vi "get_spnial_column_MD5.vi"(11 "spinal_column":T1={"Experimental Variables"={"Pixel Size before binning (µm)"=0.0, "Imaging Wavelength (m)"=0.0, "Isotope"=0, "1P1 Linewidth (MHz)"=0.0, "Imaging Detuning (MHz)"=0.0, "Software Bin Size"=0, "Exp. Trigger ON time (ms)"=0.0, "Path to spinapi.dll"=path "C:/SpinCore/SpinAPI/lib32/spinapi.dll", "PB clock_freq (MHz)"=100.0}, "Red MOT 88 Inputs"={"Active Device"="", "Active Channels"=[], "Waveform Parameters"=[], "Active Phases"=[], "Phase Times"=[], "Trigger Channel"=""}, "6713 Blue MOT"={"Active Device"="", "Active Channels"=[], "Waveform Parameters"=[], "Active Phases"=[], "Phase Times"=[], "Trigger Channel"="", "FIFO Buffer Size"=0.0, "6713_ch_labels"={"Array"=["", "", "", "", "", "", "", "", "", "", "", "", "", "", "", "", "", "", "", "", " ", "", "", ""], "PB_0_Ch_Labels\n"=["0", "1", "2", "3", "4", "5", "6", "7", "8", "9", "10", "11", "12", "13", "14", "15", "16", "17", "18", "19", "20", "21", "22", "23"]}}, "48ch_pb_array"=[], "Red MOT 87 Inputs"={"Active Device"="", "Active Channels"=[], "Waveform Parameters"=[], "Active Phases"=[], "Phase Times"=[], "Trigger Channel"=""}, "ODT Params"={"Waveform Parameters"=[], "Active Phases"=[], "Active Channels"=[], "Phase Times (s)"=[], "Active Device"="", "Trigger Channel"="", "Evaporation Phase"=0.0, "Evaporation Channel"=0.0}, "Agilent E3631A Settings"={"VISA resource name"="", "Voltage Set (6V max)"=0.0, "Current Set (5A max)"=0.0, "Voltage Set (25V max)"=0.0, "Current Set (1A max)"=0.0, "Voltage Set (-25V max)"=25.0, "Current Set (1A max)"=0.225, "6V Switch"=FALSE, "+25V Switch"=FALSE, "-25V Switch"=FALSE, "Agilent E3631A Measurements"={"6V Actual Voltage Level (V)"=0.03231557, "6V Actual Current Level (A)"=0.01701259, "25V Actual Voltage Level (V)"=0.4256878, "25V Actual Current Level (A)"=0.2772881, "-25V Actual Current Level (A)"=0.0, "-25V Actual Voltage Level (V)"=0.0}, "Triggered Agilent Settings"={"Trigger \nDelay (s)"=3.0, "Enable +6V Channel"=TRUE, "+6V Current"=0.02, "Enable -25V Channel"=FALSE, "-25V Current"=0.0, "Enable +25V Channel"=TRUE, "+25V Current"=0.275}, "Auto Program Agilent"=FALSE, "Agilent Software Trigger"=FALSE}, "PixelFly Controls"={"Acquitsition Settings"={"Buffer number"=0, "Size (Bytes)"=0, "initialized array"=array2048x1280[2621440 elements], "X Bin"=0, "Y Bin"=0, "Board Handle"=0, "Picture parameters"={"ccdxsize"=0, "ccdy"=0, "pictx"=0, "picty"=0, "bitspixel"=12}, "Buffer Out"=[]}, "Initialization"={"Exposure mode"=1, "exp time"=150, "exp level"=1, "gain"=0, "boardid in"=0, "offset"=0, "V bin"=0, "H bin"=0, "trigger"=FALSE, "Bit depth"=0}}, "Scan Parameters"={"Initial Values"=[], "Final Values"=[], "Step Sizes"=[], "Parameters to Change"=[], "Channels to Change"=[], "Number of Parameters to Scan"=0, "Parameter Nickname (no spaces)"=[], "Scan Base Name"="", "Raw_Data Folder"=path "", "ROI Parameters"={"Background Radius"=0.0, "Atom Radius"=0.0, "X Center"=0.0, "Y Center"=0.0}, "Drop Time (ms)"=0.0, "Phases To Change"=[], "Scan Pulseblaster Channel With Parameter"={"Change PB Time Toggle"=FALSE, "PB Channel"=0.0, "Parameter Number"=0.0}, "Preserve Waveform\nContinuity"=FALSE, "Generated Array Type"=enum."Custom Array From File", "Master Batch Third Column"=0.0, "Master Batch Fourth Column"=0.0, "Master Batch Fifth Column"=0.0, "Current Param. Values"=[81.5, 1.0]}, "PicoScope"={"Channel A Settings"={"Enabled"=FALSE, "Coupling"=0, "Range"=0, "Analogue Offset"=0.0}, "Channel B Settings"={"Enabled"=FALSE, "Coupling"=0, "Range"=0, "Analogue Offset"=0.0}, "Trigger Options"={"Trigger Enabled"=FALSE, "Trigger Source"=enum."Channel A", "Trigger Threshold (-5 to 5 V)"=0.0, "Trigger Slope"=0, "Trigger Delay (s)"=0.0, "Auto Trigger Time (ms)"=0}, "Pico Scope Inititalization Settings"={"USB Power"=FALSE, "Use Serial Number"=FALSE, "Resolution"=0, "Serial Number"="", "Handle"=0}, "Use PicoScope?"=FALSE, "Acquisition Settings"={"Pre Trigger Time (s)"=0.0, "Post Trigger Time (s)"=0.0, "Resolution (s)"=0.0, "Four Channel Device"=FALSE, "Number of Captures"=0.0}}, "6229 Green Lattice Inputs"={"Active Device"="", "Active Channels"=[], "Active Phases"=[], "Phase Times"=[], "Trigger Channel"="", "FIFO Buffer Size"=0.0, "Sample Step Time (us)"=0.0, "Initialization Parameters"={"Enable Initialization"=FALSE, "Initial Values"=[]}, "Waveform Parameters"=[]}, "Novatech Synth Settings"=[], "Control Reference Cluster"={"Controls[]"=[], "Control Names"=[]}, "FPGA_cntrl"={"Channel 0"={"Operation"=0, "Input A"=0, "Output - LO"=0.0, "Output - HI"=0.0, "Inputs"=[0, 0, 0, 0], "Output Values"=[0.0, 0.0, 0.0, 0.0, 0.0], "Num. Inputs"=0, "Set Point"=0.0, "Inv."=[FALSE, FALSE, FALSE, FALSE], "Inv. A"=FALSE, "Inv. B"=FALSE, "Input B"=0}, "Channel 1"={"Operation"=0, "Input A"=0, "Output - LO"=0.0, "Output - HI"=0.0, "Inputs"=[0, 0, 0, 0], "Output Values"=[0.0, 0.0, 0.0, 0.0, 0.0], "Num. Inputs"=0, "Set Point"=0.0, "Inv."=[FALSE, FALSE, FALSE, FALSE], "Inv. A"=FALSE, "Inv. B"=FALSE, "Input B"=0}, "Channel 2"={"Operation"=0, "Input A"=0, "Output - LO"=0.0, "Output - HI"=0.0, "Inputs"=[0, 0, 0, 0], "Output Values"=[0.0, 0.0, 0.0, 0.0, 0.0], "Num. Inputs"=0, "Set Point"=0.0, "Inv."=[FALSE, FALSE, FALSE, FALSE], "Inv. A"=FALSE, "Inv. B"=FALSE, "Input B"=0}, "Channel 3"={"Operation"=0, "Input A"=0, "Output - LO"=0.0, "Output - HI"=0.0, "Inputs"=[0, 0, 0, 0], "Output Values"=[0.0, 0.0, 0.0, 0.0, 0.0], "Num. Inputs"=0, "Set Point"=0.0, "Inv."=[FALSE, FALSE, FALSE, FALSE], "Inv. A"=FALSE, "Inv. B"=FALSE, "Input B"=0}, "Channel 4"={"Operation"=0, "Input A"=0, "Output - LO"=0.0, "Output - HI"=0.0, "Inputs"=[0, 0, 0, 0], "Output Values"=[0.0, 0.0, 0.0, 0.0, 0.0], "Num. Inputs"=0, "Set Point"=0.0, "Inv."=[FALSE, FALSE, FALSE, FALSE], "Inv. A"=FALSE, "Inv. B"=FALSE, "Input B"=0}, "Channel 5"={"Operation"=0, "Input A"=0, "Output - LO"=0.0, "Output - HI"=0.0, "Inputs"=[0, 0, 0, 0], "Output Values"=[0.0, 0.0, 0.0, 0.0, 0.0], "Num. Inputs"=0, "Set Point"=0.0, "Inv."=[FALSE, FALSE, FALSE, FALSE], "Inv. A"=FALSE, "Inv. B"=FALSE, "Input B"=0}, "Channel 6"={"Operation"=0, "Input A"=0, "Output - LO"=0.0, "Output - HI"=0.0, "Inputs"=[0, 0, 0, 0], "Output Values"=[0.0, 0.0, 0.0, 0.0, 0.0], "Num. Inputs"=0, "Set Point"=0.0, "Inv."=[FALSE, FALSE, FALSE, FALSE], "Inv. A"=FALSE, "Inv. B"=FALSE, "Input B"=0}, "Channel 7"={"Operation"=0, "Input A"=0, "Output - LO"=0.0, "Output - HI"=0.0, "Inputs"=[0, 0, 0, 0], "Output Values"=[0.0, 0.0, 0.0, 0.0, 0.0], "Num. Inputs"=0, "Set Point"=0.0, "Inv."=[FALSE, FALSE, FALSE, FALSE], "Inv. A"=FALSE, "Inv. B"=FALSE, "Input B"=0}, "Channel 8"={"Operation"=0, "Input A"=0, "Output - LO"=0.0, "Output - HI"=0.0, "Inputs"=[0, 0, 0, 0], "Output Values"=[0.0, 0.0, 0.0, 0.0, 0.0], "Num. Inputs"=0, "Set Point"=0.0, "Inv."=[FALSE, FALSE, FALSE, FALSE], "Inv. A"=FALSE, "Inv. B"=FALSE, "Input B"=0}, "Channel 9"={"Operation"=0, "Input A"=0, "Output - LO"=0.0, "Output - HI"=0.0, "Inputs"=[0, 0, 0, 0], "Output Values"=[0.0, 0.0, 0.0, 0.0, 0.0], "Num. Inputs"=0, "Set Point"=0.0, "Inv."=[FALSE, FALSE, FALSE, FALSE], "Inv. A"=FALSE, "Inv. B"=FALSE, "Input B"=0}, "Channel 10"={"Operation"=0, "Input A"=0, "Output - LO"=0.0, "Output - HI"=0.0, "Inputs"=[0, 0, 0, 0], "Output Values"=[0.0, 0.0, 0.0, 0.0, 0.0], "Num. Inputs"=0, "Set Point"=0.0, "Inv."=[FALSE, FALSE, FALSE, FALSE], "Inv. A"=FALSE, "Inv. B"=FALSE, "Input B"=0}, "Channel 11"={"Operation"=0, "Input A"=0, "Output - LO"=0.0, "Output - HI"=0.0, "Inputs"=[0, 0, 0, 0], "Output Values"=[0.0, 0.0, 0.0, 0.0, 0.0], "Num. Inputs"=0, "Set Point"=0.0, "Inv."=[FALSE, FALSE, FALSE, FALSE], "Inv. A"=FALSE, "Inv. B"=FALSE, "Input B"=0}, "Channel 12"={"Operation"=0, "Input A"=0, "Output - LO"=0.0, "Output - HI"=0.0, "Inputs"=[0, 0, 0, 0], "Output Values"=[0.0, 0.0, 0.0, 0.0, 0.0], "Num. Inputs"=0, "Set Point"=0.0, "Inv."=[FALSE, FALSE, FALSE, FALSE], "Inv. A"=FALSE, "Inv. B"=FALSE, "Input B"=0}, "Channel 13"={"Operation"=0, "Input A"=0, "Output - LO"=0.0, "Output - HI"=0.0, "Inputs"=[0, 0, 0, 0], "Output Values"=[0.0, 0.0, 0.0, 0.0, 0.0], "Num. Inputs"=0, "Set Point"=0.0, "Inv."=[FALSE, FALSE, FALSE, FALSE], "Inv. A"=FALSE, "Inv. B"=FALSE, "Input B"=0}, "Channel 14"={"Operation"=0, "Input A"=0, "Output - LO"=0.0, "Output - HI"=0.0, "Inputs"=[0, 0, 0, 0], "Output Values"=[0.0, 0.0, 0.0, 0.0, 0.0], "Num. Inputs"=0, "Set Point"=0.0, "Inv."=[FALSE, FALSE, FALSE, FALSE], "Inv. A"=FALSE, "Inv. B"=FALSE, "Input B"=0}, "Channel 15"={"Operation"=0, "Input A"=0, "Output - LO"=0.0, "Output - HI"=0.0, "Inputs"=[0, 0, 0, 0], "Output Values"=[0.0, 0.0, 0.0, 0.0, 0.0], "Num. Inputs"=0, "Set Point"=0.0, "Inv."=[FALSE, FALSE, FALSE, FALSE], "Inv. A"=FALSE, "Inv. B"=FALSE, "Input B"=0}}} {"Experimental Variables"."Software Bin Size" items=["1"=1, "2"=2, "3"=3, "4"=4, "5"=5, "6"=6, "7"=7, "8"=8]; "Experimental Variables"."Isotope" min=84 max=88; "Experimental Variables"."Imaging Wavelength (m)" format="%#_6p"; "Red MOT 88 Inputs"."Phase Times" format="%.0p"; "Red MOT 88 Inputs"."Waveform Parameters"."Degree" min=1.0; "6713 Blue MOT"."Phase Times" format="%.3f"; "48ch_pb_array"."Label and Instructions"."Instruct Data" format="%#.2p"; "48ch_pb_array"."Label and Instructions"."Op Code" items=["Continue", "Stop", "Loop", "End Loop", "JSR", "RTS", "Go To", "Long Delay", "Wait"]; "48ch_pb_array"."Label and Instructions"."Time (s)" min=5e-08 format="%.2p"; "Red MOT 87 Inputs"."Phase Times" format="%.0p"; "Red MOT 87 Inputs"."Waveform Parameters"."Degree" min=1.0; "ODT Params"."Evaporation Channel" min=0.0 max=1.0 step=1.0; "ODT Params"."Evaporation Phase" min=0.0 max=4.0 step=1.0; "ODT Params"."Phase Times (s)" format="%#_6p"; "Agilent E3631A Settings"."Triggered Agilent Settings"."Trigger \nDelay (s)" min=0.0 max=3600.0 step=1.0 format="%.2f"; "Agilent E3631A Settings"."Agilent E3631A Measurements"."-25V Actual Current Level (A)" format="%.3g"; "Agilent E3631A Settings"."Agilent E3631A Measurements"."-25V Actual Voltage Level (V)" format="%.3g"; "Agilent E3631A Settings"."Agilent E3631A Measurements"."25V Actual Current Level (A)" format="%.3g"; "Agilent E3631A Settings"."Agilent E3631A Measurements"."25V Actual Voltage Level (V)" format="%.3g"; "Agilent E3631A Settings"."Agilent E3631A Measurements"."6V Actual Current Level (A)" format="%.3g"; "Agilent E3631A Settings"."Agilent E3631A Measurements"."6V Actual Voltage Level (V)" format="%.3g"; "Agilent E3631A Settings"."Current Set (1A max)" format="%.3g"; "Agilent E3631A Settings"."Voltage Set (-25V max)" format="%.3g"; "Agilent E3631A Settings"."Current Set (1A max)" format="%.3g"; "Agilent E3631A Settings"."Voltage Set (25V max)" format="%.3g"; "Agilent E3631A Settings"."Current Set (5A max)" format="%.3g"; "Agilent E3631A Settings"."Voltage Set (6V max)" format="%.3g"; "PixelFly Controls"."Initialization"."Bit depth" items=["8", "12"]; "PixelFly Controls"."Initialization"."H bin" items=["1", "2"]; "PixelFly Controls"."Initialization"."V bin" items=["1", "2"]; "PixelFly Controls"."Initialization"."boardid in" min=0 max=3 step=1; "PixelFly Controls"."Initialization"."gain" items=["Low (X1)", "High (X2)"]; "PixelFly Controls"."Initialization"."exp level" min=0 max=255 step=1; "PixelFly Controls"."Initialization"."exp time" min=1 max=10000; "PixelFly Controls"."Initialization"."Exposure mode" items=["Asynch shutter", "Double shot", "Video mode", "Auto exposure"]; "Scan Parameters"."Current Param. Values" format="%^#.3e"; "Scan Parameters"."Drop Time (ms)" min=1.0; "Scan Parameters"."Number of Parameters to Scan" min=1; "PicoScope"."Acquisition Settings"."Resolution (s)" min=8e-09 max=34.36 step=8e-09 format="%#_6p"; "PicoScope"."Acquisition Settings"."Post Trigger Time (s)" min=0.0 format="%#_6p"; "PicoScope"."Acquisition Settings"."Pre Trigger Time (s)" min=0.0 format="%#_6p"; "PicoScope"."Pico Scope Inititalization Settings"."Resolution" items=["8-bit", "12-bit", "14-bit", "15-bit (max. 2 ch.)", "16-bit (max. 1 ch.)"]; "PicoScope"."Trigger Options"."Trigger Slope" items=["Rising"=2, "Falling"=3]; "PicoScope"."Channel B Settings"."Range" items=["10 mV", "20 mV", "50 mV", "100 mV", "200 mV", "500 mV", "1 V", "2 V", "5 V", "10 V", "20 V", "50 V ", "100 V"]; "PicoScope"."Channel B Settings"."Coupling" items=["AC", "DC"]; "PicoScope"."Channel A Settings"."Range" items=["10 mV", "20 mV", "50 mV", "100 mV", "200 mV", "500 mV", "1 V", "2 V", "5 V", "10 V", "20 V", "50 V ", "100 V"]; "PicoScope"."Channel A Settings"."Coupling" items=["AC", "DC"]; "6229 Green Lattice Inputs"."Phase Times" format="%_3p"; "Novatech Synth Settings"."Table Mode"."Freq. Step (MHz)" format="%#_9g"; "Novatech Synth Settings"."Table Mode"."FinalFreq" format="%#_9g"; "Novatech Synth Settings"."Table Mode"."Initial Freq.(MHz)" format="%#_9g"; "Novatech Synth Settings"."Channel Settings"."Frequency (MHz)" format="%#_9g"; "FPGA_cntrl"."Channel 15"."Input B" items=["DIO0", "DIO1", "DIO2", "DIO3", "DIO4", "DIO5", "DIO6", "DIO7", "DIO8", "DIO9", "DIO10", "DIO11", "DIO12", "DIO13", "DIO14", "DIO15", "DIO16", "DIO17", "DIO18", "DIO19", "DIO20", "DIO21", "DIO22", "DIO23", "DIO24", "DIO25", "DIO26", "DIO27", "DIO28", "DIO29", "DIO30", "DIO31", "FALSE"]; "FPGA_cntrl"."Channel 15"."Input A" items=["DIO0", "DIO1", "DIO2", "DIO3", "DIO4", "DIO5", "DIO6", "DIO7", "DIO8", "DIO9", "DIO10", "DIO11", "DIO12", "DIO13", "DIO14", "DIO15", "DIO16", "DIO17", "DIO18", "DIO19", "DIO20", "DIO21", "DIO22", "DIO23", "DIO24", "DIO25", "DIO26", "DIO27", "DIO28", "DIO29", "DIO30", "DIO31", "FALSE"]; "FPGA_cntrl"."Channel 15"."Inputs" items=["DIO0", "DIO1", "DIO2", "DIO3", "DIO4", "DIO5", "DIO6", "DIO7", "DIO8", "DIO9", "DIO10", "DIO11", "DIO12", "DIO13", "DIO14", "DIO15", "DIO16", "DIO17", "DIO18", "DIO19", "DIO20", "DIO21", "DIO22", "DIO23", "DIO24", "DIO25", "DIO26", "DIO27", "DIO28", "DIO29", "DIO30", "DIO31", "FALSE"]; "FPGA_cntrl"."Channel 15"."Operation" items=["OFF", "Constant", "Bool - Basic Switch", "Bool - AND Switch", "Bool - OR Switch", "Custom - Comp Basic Switch", "Custom - 461nm Freq."]; "FPGA_cntrl"."Channel 14"."Input B" items=["DIO0", "DIO1", "DIO2", "DIO3", "DIO4", "DIO5", "DIO6", "DIO7", "DIO8", "DIO9", "DIO10", "DIO11", "DIO12", "DIO13", "DIO14", "DIO15", "DIO16", "DIO17", "DIO18", "DIO19", "DIO20", "DIO21", "DIO22", "DIO23", "DIO24", "DIO25", "DIO26", "DIO27", "DIO28", "DIO29", "DIO30", "DIO31", "FALSE"]; "FPGA_cntrl"."Channel 14"."Input A" items=["DIO0", "DIO1", "DIO2", "DIO3", "DIO4", "DIO5", "DIO6", "DIO7", "DIO8", "DIO9", "DIO10", "DIO11", "DIO12", "DIO13", "DIO14", "DIO15", "DIO16", "DIO17", "DIO18", "DIO19", "DIO20", "DIO21", "DIO22", "DIO23", "DIO24", "DIO25", "DIO26", "DIO27", "DIO28", "DIO29", "DIO30", "DIO31", "FALSE"]; "FPGA_cntrl"."Channel 14"."Inputs" items=["DIO0", "DIO1", "DIO2", "DIO3", "DIO4", "DIO5", "DIO6", "DIO7", "DIO8", "DIO9", "DIO10", "DIO11", "DIO12", "DIO13", "DIO14", "DIO15", "DIO16", "DIO17", "DIO18", "DIO19", "DIO20", "DIO21", "DIO22", "DIO23", "DIO24", "DIO25", "DIO26", "DIO27", "DIO28", "DIO29", "DIO30", "DIO31", "FALSE"]; "FPGA_cntrl"."Channel 14"."Operation" items=["OFF", "Constant", "Bool - Basic Switch", "Bool - AND Switch", "Bool - OR Switch", "Custom - Comp Basic Switch", "Custom - 461nm Freq."]; "FPGA_cntrl"."Channel 13"."Input B" items=["DIO0", "DIO1", "DIO2", "DIO3", "DIO4", "DIO5", "DIO6", "DIO7", "DIO8", "DIO9", "DIO10", "DIO11", "DIO12", "DIO13", "DIO14", "DIO15", "DIO16", "DIO17", "DIO18", "DIO19", "DIO20", "DIO21", "DIO22", "DIO23", "DIO24", "DIO25", "DIO26", "DIO27", "DIO28", "DIO29", "DIO30", "DIO31", "FALSE"]; "FPGA_cntrl"."Channel 13"."Input A" items=["DIO0", "DIO1", "DIO2", "DIO3", "DIO4", "DIO5", "DIO6", "DIO7", "DIO8", "DIO9", "DIO10", "DIO11", "DIO12", "DIO13", "DIO14", "DIO15", "DIO16", "DIO17", "DIO18", "DIO19", "DIO20", "DIO21", "DIO22", "DIO23", "DIO24", "DIO25", "DIO26", "DIO27", "DIO28", "DIO29", "DIO30", "DIO31", "FALSE"]; "FPGA_cntrl"."Channel 13"."Inputs" items=["DIO0", "DIO1", "DIO2", "DIO3", "DIO4", "DIO5", "DIO6", "DIO7", "DIO8", "DIO9", "DIO10", "DIO11", "DIO12", "DIO13", "DIO14", "DIO15", "DIO16", "DIO17", "DIO18", "DIO19", "DIO20", "DIO21", "DIO22", "DIO23", "DIO24", "DIO25", "DIO26", "DIO27", "DIO28", "DIO29", "DIO30", "DIO31", "FALSE"]; "FPGA_cntrl"."Channel 13"."Operation" items=["OFF", "Constant", "Bool - Basic Switch", "Bool - AND Switch", "Bool - OR Switch", "Custom - Comp Basic Switch", "Custom - 461nm Freq."]; "FPGA_cntrl"."Channel 12"."Input B" items=["DIO0", "DIO1", "DIO2", "DIO3", "DIO4", "DIO5", "DIO6", "DIO7", "DIO8", "DIO9", "DIO10", "DIO11", "DIO12", "DIO13", "DIO14", "DIO15", "DIO16", "DIO17", "DIO18", "DIO19", "DIO20", "DIO21", "DIO22", "DIO23", "DIO24", "DIO25", "DIO26", "DIO27", "DIO28", "DIO29", "DIO30", "DIO31", "FALSE"]; "FPGA_cntrl"."Channel 12"."Input A" items=["DIO0", "DIO1", "DIO2", "DIO3", "DIO4", "DIO5", "DIO6", "DIO7", "DIO8", "DIO9", "DIO10", "DIO11", "DIO12", "DIO13", "DIO14", "DIO15", "DIO16", "DIO17", "DIO18", "DIO19", "DIO20", "DIO21", "DIO22", "DIO23", "DIO24", "DIO25", "DIO26", "DIO27", "DIO28", "DIO29", "DIO30", "DIO31", "FALSE"]; "FPGA_cntrl"."Channel 12"."Inputs" items=["DIO0", "DIO1", "DIO2", "DIO3", "DIO4", "DIO5", "DIO6", "DIO7", "DIO8", "DIO9", "DIO10", "DIO11", "DIO12", "DIO13", "DIO14", "DIO15", "DIO16", "DIO17", "DIO18", "DIO19", "DIO20", "DIO21", "DIO22", "DIO23", "DIO24", "DIO25", "DIO26", "DIO27", "DIO28", "DIO29", "DIO30", "DIO31", "FALSE"]; "FPGA_cntrl"."Channel 12"."Operation" items=["OFF", "Constant", "Bool - Basic Switch", "Bool - AND Switch", "Bool - OR Switch", "Custom - Comp Basic Switch", "Custom - 461nm Freq."]; "FPGA_cntrl"."Channel 11"."Input B" items=["DIO0", "DIO1", "DIO2", "DIO3", "DIO4", "DIO5", "DIO6", "DIO7", "DIO8", "DIO9", "DIO10", "DIO11", "DIO12", "DIO13", "DIO14", "DIO15", "DIO16", "DIO17", "DIO18", "DIO19", "DIO20", "DIO21", "DIO22", "DIO23", "DIO24", "DIO25", "DIO26", "DIO27", "DIO28", "DIO29", "DIO30", "DIO31", "FALSE"]; "FPGA_cntrl"."Channel 11"."Input A" items=["DIO0", "DIO1", "DIO2", "DIO3", "DIO4", "DIO5", "DIO6", "DIO7", "DIO8", "DIO9", "DIO10", "DIO11", "DIO12", "DIO13", "DIO14", "DIO15", "DIO16", "DIO17", "DIO18", "DIO19", "DIO20", "DIO21", "DIO22", "DIO23", "DIO24", "DIO25", "DIO26", "DIO27", "DIO28", "DIO29", "DIO30", "DIO31", "FALSE"]; "FPGA_cntrl"."Channel 11"."Inputs" items=["DIO0", "DIO1", "DIO2", "DIO3", "DIO4", "DIO5", "DIO6", "DIO7", "DIO8", "DIO9", "DIO10", "DIO11", "DIO12", "DIO13", "DIO14", "DIO15", "DIO16", "DIO17", "DIO18", "DIO19", "DIO20", "DIO21", "DIO22", "DIO23", "DIO24", "DIO25", "DIO26", "DIO27", "DIO28", "DIO29", "DIO30", "DIO31", "FALSE"]; "FPGA_cntrl"."Channel 11"."Operation" items=["OFF", "Constant", "Bool - Basic Switch", "Bool - AND Switch", "Bool - OR Switch", "Custom - Comp Basic Switch", "Custom - 461nm Freq."]; "FPGA_cntrl"."Channel 10"."Input B" items=["DIO0", "DIO1", "DIO2", "DIO3", "DIO4", "DIO5", "DIO6", "DIO7", "DIO8", "DIO9", "DIO10", "DIO11", "DIO12", "DIO13", "DIO14", "DIO15", "DIO16", "DIO17", "DIO18", "DIO19", "DIO20", "DIO21", "DIO22", "DIO23", "DIO24", "DIO25", "DIO26", "DIO27", "DIO28", "DIO29", "DIO30", "DIO31", "FALSE"]; "FPGA_cntrl"."Channel 10"."Input A" items=["DIO0", "DIO1", "DIO2", "DIO3", "DIO4", "DIO5", "DIO6", "DIO7", "DIO8", "DIO9", "DIO10", "DIO11", "DIO12", "DIO13", "DIO14", "DIO15", "DIO16", "DIO17", "DIO18", "DIO19", "DIO20", "DIO21", "DIO22", "DIO23", "DIO24", "DIO25", "DIO26", "DIO27", "DIO28", "DIO29", "DIO30", "DIO31", "FALSE"]; "FPGA_cntrl"."Channel 10"."Inputs" items=["DIO0", "DIO1", "DIO2", "DIO3", "DIO4", "DIO5", "DIO6", "DIO7", "DIO8", "DIO9", "DIO10", "DIO11", "DIO12", "DIO13", "DIO14", "DIO15", "DIO16", "DIO17", "DIO18", "DIO19", "DIO20", "DIO21", "DIO22", "DIO23", "DIO24", "DIO25", "DIO26", "DIO27", "DIO28", "DIO29", "DIO30", "DIO31", "FALSE"]; "FPGA_cntrl"."Channel 10"."Operation" items=["OFF", "Constant", "Bool - Basic Switch", "Bool - AND Switch", "Bool - OR Switch", "Custom - Comp Basic Switch", "Custom - 461nm Freq."]; "FPGA_cntrl"."Channel 9"."Input B" items=["DIO0", "DIO1", "DIO2", "DIO3", "DIO4", "DIO5", "DIO6", "DIO7", "DIO8", "DIO9", "DIO10", "DIO11", "DIO12", "DIO13", "DIO14", "DIO15", "DIO16", "DIO17", "DIO18", "DIO19", "DIO20", "DIO21", "DIO22", "DIO23", "DIO24", "DIO25", "DIO26", "DIO27", "DIO28", "DIO29", "DIO30", "DIO31", "FALSE"]; "FPGA_cntrl"."Channel 9"."Input A" items=["DIO0", "DIO1", "DIO2", "DIO3", "DIO4", "DIO5", "DIO6", "DIO7", "DIO8", "DIO9", "DIO10", "DIO11", "DIO12", "DIO13", "DIO14", "DIO15", "DIO16", "DIO17", "DIO18", "DIO19", "DIO20", "DIO21", "DIO22", "DIO23", "DIO24", "DIO25", "DIO26", "DIO27", "DIO28", "DIO29", "DIO30", "DIO31", "FALSE"]; "FPGA_cntrl"."Channel 9"."Inputs" items=["DIO0", "DIO1", "DIO2", "DIO3", "DIO4", "DIO5", "DIO6", "DIO7", "DIO8", "DIO9", "DIO10", "DIO11", "DIO12", "DIO13", "DIO14", "DIO15", "DIO16", "DIO17", "DIO18", "DIO19", "DIO20", "DIO21", "DIO22", "DIO23", "DIO24", "DIO25", "DIO26", "DIO27", "DIO28", "DIO29", "DIO30", "DIO31", "FALSE"]; "FPGA_cntrl"."Channel 9"."Operation" items=["OFF", "Constant", "Bool - Basic Switch", "Bool - AND Switch", "Bool - OR Switch", "Custom - Comp Basic Switch", "Custom - 461nm Freq."]; "FPGA_cntrl"."Channel 8"."Input B" items=["DIO0", "DIO1", "DIO2", "DIO3", "DIO4", "DIO5", "DIO6", "DIO7", "DIO8", "DIO9", "DIO10", "DIO11", "DIO12", "DIO13", "DIO14", "DIO15", "DIO16", "DIO17", "DIO18", "DIO19", "DIO20", "DIO21", "DIO22", "DIO23", "DIO24", "DIO25", "DIO26", "DIO27", "DIO28", "DIO29", "DIO30", "DIO31", "FALSE"]; "FPGA_cntrl"."Channel 8"."Input A" items=["DIO0", "DIO1", "DIO2", "DIO3", "DIO4", "DIO5", "DIO6", "DIO7", "DIO8", "DIO9", "DIO10", "DIO11", "DIO12", "DIO13", "DIO14", "DIO15", "DIO16", "DIO17", "DIO18", "DIO19", "DIO20", "DIO21", "DIO22", "DIO23", "DIO24", "DIO25", "DIO26", "DIO27", "DIO28", "DIO29", "DIO30", "DIO31", "FALSE"]; "FPGA_cntrl"."Channel 8"."Inputs" items=["DIO0", "DIO1", "DIO2", "DIO3", "DIO4", "DIO5", "DIO6", "DIO7", "DIO8", "DIO9", "DIO10", "DIO11", "DIO12", "DIO13", "DIO14", "DIO15", "DIO16", "DIO17", "DIO18", "DIO19", "DIO20", "DIO21", "DIO22", "DIO23", "DIO24", "DIO25", "DIO26", "DIO27", "DIO28", "DIO29", "DIO30", "DIO31", "FALSE"]; "FPGA_cntrl"."Channel 8"."Operation" items=["OFF", "Constant", "Bool - Basic Switch", "Bool - AND Switch", "Bool - OR Switch", "Custom - Comp Basic Switch", "Custom - 461nm Freq."]; "FPGA_cntrl"."Channel 7"."Input B" items=["DIO0", "DIO1", "DIO2", "DIO3", "DIO4", "DIO5", "DIO6", "DIO7", "DIO8", "DIO9", "DIO10", "DIO11", "DIO12", "DIO13", "DIO14", "DIO15", "DIO16", "DIO17", "DIO18", "DIO19", "DIO20", "DIO21", "DIO22", "DIO23", "DIO24", "DIO25", "DIO26", "DIO27", "DIO28", "DIO29", "DIO30", "DIO31", "FALSE"]; "FPGA_cntrl"."Channel 7"."Input A" items=["DIO0", "DIO1", "DIO2", "DIO3", "DIO4", "DIO5", "DIO6", "DIO7", "DIO8", "DIO9", "DIO10", "DIO11", "DIO12", "DIO13", "DIO14", "DIO15", "DIO16", "DIO17", "DIO18", "DIO19", "DIO20", "DIO21", "DIO22", "DIO23", "DIO24", "DIO25", "DIO26", "DIO27", "DIO28", "DIO29", "DIO30", "DIO31", "FALSE"]; "FPGA_cntrl"."Channel 7"."Inputs" items=["DIO0", "DIO1", "DIO2", "DIO3", "DIO4", "DIO5", "DIO6", "DIO7", "DIO8", "DIO9", "DIO10", "DIO11", "DIO12", "DIO13", "DIO14", "DIO15", "DIO16", "DIO17", "DIO18", "DIO19", "DIO20", "DIO21", "DIO22", "DIO23", "DIO24", "DIO25", "DIO26", "DIO27", "DIO28", "DIO29", "DIO30", "DIO31", "FALSE"]; "FPGA_cntrl"."Channel 7"."Operation" items=["OFF", "Constant", "Bool - Basic Switch", "Bool - AND Switch", "Bool - OR Switch", "Custom - Comp Basic Switch", "Custom - 461nm Freq."]; "FPGA_cntrl"."Channel 6"."Input B" items=["DIO0", "DIO1", "DIO2", "DIO3", "DIO4", "DIO5", "DIO6", "DIO7", "DIO8", "DIO9", "DIO10", "DIO11", "DIO12", "DIO13", "DIO14", "DIO15", "DIO16", "DIO17", "DIO18", "DIO19", "DIO20", "DIO21", "DIO22", "DIO23", "DIO24", "DIO25", "DIO26", "DIO27", "DIO28", "DIO29", "DIO30", "DIO31", "FALSE"]; "FPGA_cntrl"."Channel 6"."Input A" items=["DIO0", "DIO1", "DIO2", "DIO3", "DIO4", "DIO5", "DIO6", "DIO7", "DIO8", "DIO9", "DIO10", "DIO11", "DIO12", "DIO13", "DIO14", "DIO15", "DIO16", "DIO17", "DIO18", "DIO19", "DIO20", "DIO21", "DIO22", "DIO23", "DIO24", "DIO25", "DIO26", "DIO27", "DIO28", "DIO29", "DIO30", "DIO31", "FALSE"]; "FPGA_cntrl"."Channel 6"."Inputs" items=["DIO0", "DIO1", "DIO2", "DIO3", "DIO4", "DIO5", "DIO6", "DIO7", "DIO8", "DIO9", "DIO10", "DIO11", "DIO12", "DIO13", "DIO14", "DIO15", "DIO16", "DIO17", "DIO18", "DIO19", "DIO20", "DIO21", "DIO22", "DIO23", "DIO24", "DIO25", "DIO26", "DIO27", "DIO28", "DIO29", "DIO30", "DIO31", "FALSE"]; "FPGA_cntrl"."Channel 6"."Operation" items=["OFF", "Constant", "Bool - Basic Switch", "Bool - AND Switch", "Bool - OR Switch", "Custom - Comp Basic Switch", "Custom - 461nm Freq."]; "FPGA_cntrl"."Channel 5"."Input B" items=["DIO0", "DIO1", "DIO2", "DIO3", "DIO4", "DIO5", "DIO6", "DIO7", "DIO8", "DIO9", "DIO10", "DIO11", "DIO12", "DIO13", "DIO14", "DIO15", "DIO16", "DIO17", "DIO18", "DIO19", "DIO20", "DIO21", "DIO22", "DIO23", "DIO24", "DIO25", "DIO26", "DIO27", "DIO28", "DIO29", "DIO30", "DIO31", "FALSE"]; "FPGA_cntrl"."Channel 5"."Input A" items=["DIO0", "DIO1", "DIO2", "DIO3", "DIO4", "DIO5", "DIO6", "DIO7", "DIO8", "DIO9", "DIO10", "DIO11", "DIO12", "DIO13", "DIO14", "DIO15", "DIO16", "DIO17", "DIO18", "DIO19", "DIO20", "DIO21", "DIO22", "DIO23", "DIO24", "DIO25", "DIO26", "DIO27", "DIO28", "DIO29", "DIO30", "DIO31", "FALSE"]; "FPGA_cntrl"."Channel 5"."Inputs" items=["DIO0", "DIO1", "DIO2", "DIO3", "DIO4", "DIO5", "DIO6", "DIO7", "DIO8", "DIO9", "DIO10", "DIO11", "DIO12", "DIO13", "DIO14", "DIO15", "DIO16", "DIO17", "DIO18", "DIO19", "DIO20", "DIO21", "DIO22", "DIO23", "DIO24", "DIO25", "DIO26", "DIO27", "DIO28", "DIO29", "DIO30", "DIO31", "FALSE"]; "FPGA_cntrl"."Channel 5"."Operation" items=["OFF", "Constant", "Bool - Basic Switch", "Bool - AND Switch", "Bool - OR Switch", "Custom - Comp Basic Switch", "Custom - 461nm Freq."]; "FPGA_cntrl"."Channel 4"."Input B" items=["DIO0", "DIO1", "DIO2", "DIO3", "DIO4", "DIO5", "DIO6", "DIO7", "DIO8", "DIO9", "DIO10", "DIO11", "DIO12", "DIO13", "DIO14", "DIO15", "DIO16", "DIO17", "DIO18", "DIO19", "DIO20", "DIO21", "DIO22", "DIO23", "DIO24", "DIO25", "DIO26", "DIO27", "DIO28", "DIO29", "DIO30", "DIO31", "FALSE"]; "FPGA_cntrl"."Channel 4"."Input A" items=["DIO0", "DIO1", "DIO2", "DIO3", "DIO4", "DIO5", "DIO6", "DIO7", "DIO8", "DIO9", "DIO10", "DIO11", "DIO12", "DIO13", "DIO14", "DIO15", "DIO16", "DIO17", "DIO18", "DIO19", "DIO20", "DIO21", "DIO22", "DIO23", "DIO24", "DIO25", "DIO26", "DIO27", "DIO28", "DIO29", "DIO30", "DIO31", "FALSE"]; "FPGA_cntrl"."Channel 4"."Inputs" items=["DIO0", "DIO1", "DIO2", "DIO3", "DIO4", "DIO5", "DIO6", "DIO7", "DIO8", "DIO9", "DIO10", "DIO11", "DIO12", "DIO13", "DIO14", "DIO15", "DIO16", "DIO17", "DIO18", "DIO19", "DIO20", "DIO21", "DIO22", "DIO23", "DIO24", "DIO25", "DIO26", "DIO27", "DIO28", "DIO29", "DIO30", "DIO31", "FALSE"]; "FPGA_cntrl"."Channel 4"."Operation" items=["OFF", "Constant", "Bool - Basic Switch", "Bool - AND Switch", "Bool - OR Switch", "Custom - Comp Basic Switch", "Custom - 461nm Freq."]; "FPGA_cntrl"."Channel 3"."Input B" items=["DIO0", "DIO1", "DIO2", "DIO3", "DIO4", "DIO5", "DIO6", "DIO7", "DIO8", "DIO9", "DIO10", "DIO11", "DIO12", "DIO13", "DIO14", "DIO15", "DIO16", "DIO17", "DIO18", "DIO19", "DIO20", "DIO21", "DIO22", "DIO23", "DIO24", "DIO25", "DIO26", "DIO27", "DIO28", "DIO29", "DIO30", "DIO31", "FALSE"]; "FPGA_cntrl"."Channel 3"."Input A" items=["DIO0", "DIO1", "DIO2", "DIO3", "DIO4", "DIO5", "DIO6", "DIO7", "DIO8", "DIO9", "DIO10", "DIO11", "DIO12", "DIO13", "DIO14", "DIO15", "DIO16", "DIO17", "DIO18", "DIO19", "DIO20", "DIO21", "DIO22", "DIO23", "DIO24", "DIO25", "DIO26", "DIO27", "DIO28", "DIO29", "DIO30", "DIO31", "FALSE"]; "FPGA_cntrl"."Channel 3"."Inputs" items=["DIO0", "DIO1", "DIO2", "DIO3", "DIO4", "DIO5", "DIO6", "DIO7", "DIO8", "DIO9", "DIO10", "DIO11", "DIO12", "DIO13", "DIO14", "DIO15", "DIO16", "DIO17", "DIO18", "DIO19", "DIO20", "DIO21", "DIO22", "DIO23", "DIO24", "DIO25", "DIO26", "DIO27", "DIO28", "DIO29", "DIO30", "DIO31", "FALSE"]; "FPGA_cntrl"."Channel 3"."Operation" items=["OFF", "Constant", "Bool - Basic Switch", "Bool - AND Switch", "Bool - OR Switch", "Custom - Comp Basic Switch", "Custom - 461nm Freq."]; "FPGA_cntrl"."Channel 2"."Input B" items=["DIO0", "DIO1", "DIO2", "DIO3", "DIO4", "DIO5", "DIO6", "DIO7", "DIO8", "DIO9", "DIO10", "DIO11", "DIO12", "DIO13", "DIO14", "DIO15", "DIO16", "DIO17", "DIO18", "DIO19", "DIO20", "DIO21", "DIO22", "DIO23", "DIO24", "DIO25", "DIO26", "DIO27", "DIO28", "DIO29", "DIO30", "DIO31", "FALSE"]; "FPGA_cntrl"."Channel 2"."Input A" items=["DIO0", "DIO1", "DIO2", "DIO3", "DIO4", "DIO5", "DIO6", "DIO7", "DIO8", "DIO9", "DIO10", "DIO11", "DIO12", "DIO13", "DIO14", "DIO15", "DIO16", "DIO17", "DIO18", "DIO19", "DIO20", "DIO21", "DIO22", "DIO23", "DIO24", "DIO25", "DIO26", "DIO27", "DIO28", "DIO29", "DIO30", "DIO31", "FALSE"]; "FPGA_cntrl"."Channel 2"."Inputs" items=["DIO0", "DIO1", "DIO2", "DIO3", "DIO4", "DIO5", "DIO6", "DIO7", "DIO8", "DIO9", "DIO10", "DIO11", "DIO12", "DIO13", "DIO14", "DIO15", "DIO16", "DIO17", "DIO18", "DIO19", "DIO20", "DIO21", "DIO22", "DIO23", "DIO24", "DIO25", "DIO26", "DIO27", "DIO28", "DIO29", "DIO30", "DIO31", "FALSE"]; "FPGA_cntrl"."Channel 2"."Operation" items=["OFF", "Constant", "Bool - Basic Switch", "Bool - AND Switch", "Bool - OR Switch", "Custom - Comp Basic Switch", "Custom - 461nm Freq."]; "FPGA_cntrl"."Channel 1"."Input B" items=["DIO0", "DIO1", "DIO2", "DIO3", "DIO4", "DIO5", "DIO6", "DIO7", "DIO8", "DIO9", "DIO10", "DIO11", "DIO12", "DIO13", "DIO14", "DIO15", "DIO16", "DIO17", "DIO18", "DIO19", "DIO20", "DIO21", "DIO22", "DIO23", "DIO24", "DIO25", "DIO26", "DIO27", "DIO28", "DIO29", "DIO30", "DIO31", "FALSE"]; "FPGA_cntrl"."Channel 1"."Input A" items=["DIO0", "DIO1", "DIO2", "DIO3", "DIO4", "DIO5", "DIO6", "DIO7", "DIO8", "DIO9", "DIO10", "DIO11", "DIO12", "DIO13", "DIO14", "DIO15", "DIO16", "DIO17", "DIO18", "DIO19", "DIO20", "DIO21", "DIO22", "DIO23", "DIO24", "DIO25", "DIO26", "DIO27", "DIO28", "DIO29", "DIO30", "DIO31", "FALSE"]; "FPGA_cntrl"."Channel 1"."Inputs" items=["DIO0", "DIO1", "DIO2", "DIO3", "DIO4", "DIO5", "DIO6", "DIO7", "DIO8", "DIO9", "DIO10", "DIO11", "DIO12", "DIO13", "DIO14", "DIO15", "DIO16", "DIO17", "DIO18", "DIO19", "DIO20", "DIO21", "DIO22", "DIO23", "DIO24", "DIO25", "DIO26", "DIO27", "DIO28", "DIO29", "DIO30", "DIO31", "FALSE"]; "FPGA_cntrl"."Channel 1"."Operation" items=["OFF", "Constant", "Bool - Basic Switch", "Bool - AND Switch", "Bool - OR Switch", "Custom - Comp Basic Switch", "Custom - 461nm Freq."]; "FPGA_cntrl"."Channel 0"."Input B" items=["DIO0", "DIO1", "DIO2", "DIO3", "DIO4", "DIO5", "DIO6", "DIO7", "DIO8", "DIO9", "DIO10", "DIO11", "DIO12", "DIO13", "DIO14", "DIO15", "DIO16", "DIO17", "DIO18", "DIO19", "DIO20", "DIO21", "DIO22", "DIO23", "DIO24", "DIO25", "DIO26", "DIO27", "DIO28", "DIO29", "DIO30", "DIO31", "FALSE"]; "FPGA_cntrl"."Channel 0"."Input A" items=["DIO0", "DIO1", "DIO2", "DIO3", "DIO4", "DIO5", "DIO6", "DIO7", "DIO8", "DIO9", "DIO10", "DIO11", "DIO12", "DIO13", "DIO14", "DIO15", "DIO16", "DIO17", "DIO18", "DIO19", "DIO20", "DIO21", "DIO22", "DIO23", "DIO24", "DIO25", "DIO26", "DIO27", "DIO28", "DIO29", "DIO30", "DIO31", "FALSE"]; "FPGA_cntrl"."Channel 0"."Inputs" items=["DIO0", "DIO1", "DIO2", "DIO3", "DIO4", "DIO5", "DIO6", "DIO7", "DIO8", "DIO9", "DIO10", "DIO11", "DIO12", "DIO13", "DIO14", "DIO15", "DIO16", "DIO17", "DIO18", "DIO19", "DIO20", "DIO21", "DIO22", "DIO23", "DIO24", "DIO25", "DIO26", "DIO27", "DIO28", "DIO29", "DIO30", "DIO31", "FALSE"]; "FPGA_cntrl"."Channel 0"."Operation" items=["OFF", "Constant", "Bool - Basic Switch", "Bool - AND Switch", "Bool - OR Switch", "Custom - Comp Basic Switch", "Custom - 461nm Freq."]}) -> (3 "current spinal_column MD5":string)   [LabVIEW 2016]
uses:
  Controls/Spinal Column/spinal_column.ctl
  Controls/ExperimentParameters/experimentalvariables.ctl
  6733_Red_MOT/6733_control_panel.ctl
  6733_Red_MOT/6733_waveform_parameter_array.ctl
  6733_Red_MOT/6733_waveform_item.ctl
  6733_Red_MOT/Neutral_voltage_conversion_control.ctl
  Controls/6733/Trigger_Channel_Selector.ctl
  Controls/6713/6713_waveform_generation.ctl
  Controls/6713/6713_waveform_parameter_array.ctl
  Controls/6713/6713_static_waveform_item.ctl
  Controls/6713/6713_ch_labels.ctl
  Controls/PulseBlaster/48ch_pb_array.ctl
  Controls/PulseBlaster/48ch_single_timing_column_condensed.ctl
  Neutral_DAQ/6221 arb waveforms/6221_panel.ctl
  Controls/6221/6221_waveform_input.ctl
  Neutral_DAQ/6221 arb waveforms/6221_waveform_param.ctl
  Controls/Agilent E3631A/Settings_Control.ctl
  Controls/Agilent E3631A/Measurement_Indicator.ctl
  Controls/Agilent E3631A/Trigger_Settings.ctl
  Controls/PixelFly/PixelFly_Control.ctl
  Controls/PixelFly/Acquisition Settings.ctl
  Controls/PixelFly/Bit_Depth_Enum.ctl
  Controls/ScanParameters/ScanParametersPanel.ctl
  Controls/ScanParameters/ParameterToChange.ctl
  Controls/ScanParameters/ROI_set.ctl
  Controls/ScanParameters/ScanPBandParam.ctl
  Controls/PicoScope/pico_control_panel.ctl
  Controls/PicoScope/pico_channel_settings.ctl
  Controls/PicoScope/pico_trigger.ctl
  Controls/PicoScope/pico_init_settings.ctl
  Controls/6229/6229_arb_waveform_generation.ctl
  Controls/6229/6229_evap_waveform_input.ctl
  Controls/Synth_409b/Synth_controls.ctl
  Controls/Synth_409b/synth_channel.ctl
  Controls/Synth_409b/table_mode.ctl
  FPGA Control System/multiFuncProj-v2/op_ctrl_cluster.ctl
  FPGA Control System/multiFuncProj-v2/op_ctrl_element.ctl
  FPGA Control System/multiFuncProj-v2/DIO_selector.ctl
  FPGA Control System/multiFuncProj-v2/output_value.ctl
  <vilib>/Utility/Data Type/NI_Data Type.lvlib
panel:
  # "Since the Agilent is slow to communicate the program will skip programming if the \"Auto Program Agilent\" switch is disabled.  If \"Auto Program\" is enabled the settings to the far left are used to program the Agilent.\n\nAdditionally, the Agilent has an internal software trigger that can a single channel between two current setpoints. The clock is not referenced to the Pulseblaster so be careful with timing when using the Triggered Agilent Settings. To enabled this mode use the \"Agilent Software Trigger\" swithc.\n\nUse the \"Program Agilent\" button to perform a one-time write (with settings on the far left) to avoid having the slow response of the supply during data scans.\n\nNOTE: When setting only current values the program will default to setting the maximum allowed voltage for a given channel."
  # "6V (2017.06.15)\n\nReported Current = \nSet Cur - 0.003A\n\nActual Current = \nSet Cur - 0.0015A"
  # "+25V (2017.06.15)\n\nReported Current = \nSet Cur + 0.002A\n\nActual Current = \nSet Cur + 0.002A"
  # "-25V (2017.06.15)\n\nReported Current = \nSet Cur\n\nActual Current = \nSet Cur"
  # "Beware of the offset in set, reported and actual current from Agilent channels. Below are corrections measured for each channel"
  # "--25V  Measurements"
  # "+25V  Measurements"
  # "6V  Measurements"
  # "-25V Output Settings"
  # "+25V Output Settings"
  # "6V Output Settings"
  # "Select a PB Channel to set with a phase time for evaporation or whatever"
  # "(0) Arm A"
  # "(1) Arm B"
  # "(2) Arm C"
  # "(3) Unused"
  # "(0) Arm A"
  # "(1) Arm B"
  # "(2) Arm C"
  # "(3) Unused"
  # "Constant Operation Control"
  # "Boolean Operation Control"
  # "Custom Operation Controls"
  # "Constant Operation Control"
  # "Boolean Operation Control"
  # "Custom Operation Controls"
  # "Constant Operation Control"
  # "Boolean Operation Control"
  # "Custom Operation Controls"
  # "Constant Operation Control"
  # "Boolean Operation Control"
  # "Custom Operation Controls"
  # "Constant Operation Control"
  # "Boolean Operation Control"
  # "Custom Operation Controls"
  # "Constant Operation Control"
  # "Boolean Operation Control"
  # "Custom Operation Controls"
  # "Constant Operation Control"
  # "Boolean Operation Control"
  # "Custom Operation Controls"
  # "Constant Operation Control"
  # "Boolean Operation Control"
  # "Custom Operation Controls"
  # "Constant Operation Control"
  # "Boolean Operation Control"
  # "Custom Operation Controls"
  # "Constant Operation Control"
  # "Boolean Operation Control"
  # "Custom Operation Controls"
  # "Constant Operation Control"
  # "Boolean Operation Control"
  # "Custom Operation Controls"
  # "Constant Operation Control"
  # "Boolean Operation Control"
  # "Custom Operation Controls"
  # "Constant Operation Control"
  # "Boolean Operation Control"
  # "Custom Operation Controls"
  # "Constant Operation Control"
  # "Boolean Operation Control"
  # "Custom Operation Controls"
  # "Constant Operation Control"
  # "Boolean Operation Control"
  # "Custom Operation Controls"
  # "Constant Operation Control"
  # "Boolean Operation Control"
  # "Custom Operation Controls"
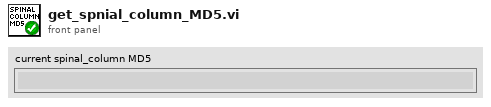
[diagram p1: front panel]
types:
  T1 = typedef "spinal_column.ctl" = cluster{"Experimental Variables":T2, "Red MOT 88 Inputs":T3, "6713 Blue MOT":T8, "48ch_pb_array":T12, "Red MOT 87 Inputs":T3, "ODT Params":T14, "Agilent E3631A Settings":T17, "PixelFly Controls":T20, "Scan Parameters":T23, "PicoScope":T27, "6229 Green Lattice Inputs":T31, "Novatech Synth Settings":T33[][], "Control Reference Cluster":cluster{"Controls[]":refnum<vi>[], "Control Names":string[]}, "FPGA_cntrl":T36}
  T2 = typedef "experimentalvariables.ctl" = cluster{"Pixel Size before binning (µm)":dbl, "Imaging Wavelength (m)":dbl, "Isotope":i32, "1P1 Linewidth (MHz)":dbl, "Imaging Detuning (MHz)":dbl, "Software Bin Size":u16, "Exp. Trigger ON time (ms)":dbl, "Path to spinapi.dll":path, "PB clock_freq (MHz)":dbl}
  T3 = typedef "6733_control_panel.ctl" = cluster{"Active Device":string, "Active Channels":bool[], "Waveform Parameters":T4, "Active Phases":bool[], "Phase Times":dbl[], "Trigger Channel":T7}
  T4 = typedef "6733_waveform_parameter_array.ctl" = T5[][]
  T5 = typedef "6733_waveform_item.ctl" = cluster{"Function":enum16{"Polynomial", "Exponential", "Constant", "Tanh"}, "Initial":dbl, "Final":dbl, "Degree":dbl, "Nickname":string, "Conversion":T6, "Constant":dbl}
  T6 = typedef "Neutral_voltage_conversion_control.ctl" = enum16{"Volts", "B Field Grad (G/cm)", "Red Boson Cntr Freq (MHz)", "Red Boson Dither Amp (kHz)", "Red Boson Power (mW)", "Red 87 Trap Cntr Freq (MHz)", "Red 87 Trap Dither Amp (kHz)", "Red 87 Trap Power (mW)", "Red 87 Stir Cntr Freq (MHz)", "Red 87 Stir Dither Amp (kHz)", "Red 87 Stir Power (mW)", "ODT Sheet Trap Power (W)", "ODT Loading Trap Power (W)"}
  T7 = typedef "Trigger_Channel_Selector.ctl" = tag
  T8 = typedef "6713_waveform_generation.ctl" = cluster{"Active Device":string, "Active Channels":bool[], "Waveform Parameters":T9, "Active Phases":bool[], "Phase Times":dbl[], "Trigger Channel":tag, "FIFO Buffer Size":dbl, "6713_ch_labels":T11}
  T9 = typedef "6713_waveform_parameter_array.ctl" = T10[][]
  T10 = typedef "6713_static_waveform_item.ctl" = cluster{"Constant":dbl, "Nickname":string, "Conversion":T6}
  T11 = typedef "6713_ch_labels.ctl" = cluster{"Array":string[], "PB_0_Ch_Labels\n":string[]}
  T12 = typedef "48ch_pb_array.ctl" = T13[]
  T13 = typedef "48ch_single_timing_column_condensed.ctl" = cluster{"Label and Instructions":cluster{"Column Number":string, "Comments":string, "Time (s)        ":dbl, "Op Code":i32, "Instruct Data":i32}, "PB_1_Bools":bool[], "Column Number":string, "Column Number 2":string, "PB_0_Bools":bool[], "Ch_Labels":string[]}
  T14 = typedef "6221_panel.ctl" = cluster{"Waveform Parameters":T15, "Active Phases":bool[], "Active Channels":bool[], "Phase Times (s)":dbl[], "Active Device":string, "Trigger Channel":tag, "Evaporation Phase":dbl, "Evaporation Channel":dbl}
  T15 = typedef "6221_waveform_input.ctl" = T16[][]
  T16 = typedef "6221_waveform_param.ctl" = cluster{"Initial Value":dbl, "Final Value":dbl, "Tau":dbl, "Eta":dbl, "Nickname":string, "Function Type":enum16{"Constant", "Power Law", "Evap - Calc Tau", "Evaporation Formula", "Tanh", "Exponential"}, "Conversion":T6, "Constant":dbl}
  T17 = typedef "Settings_Control.ctl" = cluster{"VISA resource name":refnum<visa-resource-name>, "Voltage Set (6V max)":dbl, "Current Set (5A max)":dbl, "Voltage Set (25V max)":dbl, "Current Set (1A max)":dbl, "Voltage Set (-25V max)":dbl, "Current Set (1A max)":dbl, "6V Switch":bool, "+25V Switch":bool, "-25V Switch":bool, "Agilent E3631A Measurements":T18, "Triggered Agilent Settings":T19, "Auto Program Agilent":bool, "Agilent Software Trigger":bool}
  T18 = typedef "Measurement_Indicator.ctl" = cluster{"6V Actual Voltage Level (V)":dbl, "6V Actual Current Level (A)":dbl, "25V Actual Voltage Level (V)":dbl, "25V Actual Current Level (A)":dbl, "-25V Actual Current Level (A)":dbl, "-25V Actual Voltage Level (V)":dbl}
  T19 = typedef "Trigger_Settings.ctl" = cluster{"Trigger \nDelay (s)":dbl, "Enable +6V Channel":bool, "+6V Current":dbl, "Enable -25V Channel":bool, "-25V Current":dbl, "Enable +25V Channel":bool, "+25V Current":dbl}
  T20 = typedef "PixelFly_Control.ctl" = cluster{"Acquitsition Settings":T21, "Initialization":cluster{"Exposure mode":u16, "exp time":i32, "exp level":i32, "gain":i32, "boardid in":i32, "offset":i32, "V bin":i32, "H bin":i32, "trigger":bool, "Bit depth":T22}}
  T21 = typedef "Acquisition Settings.ctl" = cluster{"Buffer number":i32, "Size (Bytes)":i32, "initialized array":u16[][], "X Bin":i32, "Y Bin":i32, "Board Handle":u32, "Picture parameters":cluster{"ccdxsize":i32, "ccdy":i32, "pictx":i32, "picty":i32, "bitspixel":i32}, "Buffer Out":u16[]}
  T22 = typedef "Bit_Depth_Enum.ctl" = i32
  T23 = typedef "ScanParametersPanel.ctl" = cluster{"Initial Values":dbl[], "Final Values":dbl[], "Step Sizes":dbl[], "Parameters to Change":T24[], "Channels to Change":u32[], "Number of Parameters to Scan":i32, "Parameter Nickname (no spaces)":string[], "Scan Base Name":string, "Raw_Data Folder":path, "ROI Parameters":T25, "Drop Time (ms)":dbl, "Phases To Change":u32[], "Scan Pulseblaster Channel With Parameter":T26, "Preserve Waveform\nContinuity":bool, "Generated Array Type":enum16{"Custom Array From File", "Default (old way)"}, "Master Batch Third Column":dbl, "Master Batch Fourth Column":dbl, "Master Batch Fifth Column":dbl, "Current Param. Values":dbl[]}
  T24 = typedef "ParameterToChange.ctl" = enum16{"Dummy Variable", "Synth Amplitude", "Synth Frequency", "Synth Phase", "ODT Params Phase Time", "ODT Params Tau", "ODT Params Final Voltage", "ODT Params Initial Voltage", "ODT Params Eta", "Red Mot 88 Phase Time", "Red Mot 87 Phase Time", "Red Mot 88 Final Voltage", "Red Mot 88 Initial Voltage", "Red Mot 87 Final Voltage", "Red Mot 87 Initial Voltage", "PulseBlaster", "6713 Voltage", "Green Lattice Phase Time", "Green Lattice Initial Voltage", "Green Lattice Final Voltage", "Agilent Current Setpoint", "FPGA - Constant Op - Set", "FPGA - Bool Op - Output HI", "FPGA - Bool Op - Output LO", "FPGA - Custom Op"}
  T25 = typedef "ROI_set.ctl" = cluster{"Background Radius":dbl, "Atom Radius":dbl, "X Center":dbl, "Y Center":dbl}
  T26 = typedef "ScanPBandParam.ctl" = cluster{"Change PB Time Toggle":bool, "PB Channel":dbl, "Parameter Number":dbl}
  T27 = typedef "pico_control_panel.ctl" = cluster{"Channel A Settings":T28, "Channel B Settings":T28, "Trigger Options":T29, "Pico Scope Inititalization Settings":T30, "Use PicoScope?":bool, "Acquisition Settings":cluster{"Pre Trigger Time (s)":dbl, "Post Trigger Time (s)":dbl, "Resolution (s)":dbl, "Four Channel Device":bool, "Number of Captures":dbl}}
  T28 = typedef "pico_channel_settings.ctl" = cluster{"Enabled":bool, "Coupling":i16, "Range":u16, "Analogue Offset":sgl}
  T29 = typedef "pico_trigger.ctl" = cluster{"Trigger Enabled":bool, "Trigger Source":enum16{"Channel A", "Channel B", "Channel C", "Channel D", "Ext."}, "Trigger Threshold (-5 to 5 V)":dbl, "Trigger Slope":u16, "Trigger Delay (s)":dbl, "Auto Trigger Time (ms)":i16}
  T30 = typedef "pico_init_settings.ctl" = cluster{"USB Power":bool, "Use Serial Number":bool, "Resolution":i32, "Serial Number":string, "Handle":i16}
  T31 = typedef "6229_arb_waveform_generation.ctl" = cluster{"Active Device":string, "Active Channels":bool[], "Active Phases":bool[], "Phase Times":dbl[], "Trigger Channel":tag, "FIFO Buffer Size":dbl, "Sample Step Time (us)":dbl, "Initialization Parameters":cluster{"Enable Initialization":bool, "Initial Values":dbl[]}, "Waveform Parameters":T32}
  T32 = typedef "6229_evap_waveform_input.ctl" = T16[][]
  T33 = typedef "Synth_controls.ctl" = cluster{"Channel Settings":T34[], "Active Chans":bool[], "COM Port":refnum<visa-resource-name>, "Table Mode":T35}
  T34 = typedef "synth_channel.ctl" = cluster{"Voltage (Amp.) ":dbl, "Frequency (MHz)":dbl, "Phase (deg)":dbl, "Nickname":string}
  T35 = typedef "table_mode.ctl" = cluster{"Initial Freq.(MHz)":dbl, "FinalFreq":dbl, "Freq. Step (MHz)":dbl, "Voltage (Amp.)":dbl, "Asc. & Desc.":bool, "Custom Frequencies":dbl[], "Custom Amplitude":dbl[], "Table Mode Switch":bool, "Array Gen":enum16{"Auto", "Custom"}, "Randomize":bool, "Continuous":bool}
  T36 = typedef "op_ctrl_cluster.ctl" = cluster{"Channel 0":T37, "Channel 1":T37, "Channel 2":T37, "Channel 3":T37, "Channel 4":T37, "Channel 5":T37, "Channel 6":T37, "Channel 7":T37, "Channel 8":T37, "Channel 9":T37, "Channel 10":T37, "Channel 11":T37, "Channel 12":T37, "Channel 13":T37, "Channel 14":T37, "Channel 15":T37}
  T37 = typedef "op_ctrl_element.ctl" = cluster{"Operation":i16, "Input A":T38, "Output - LO":T39, "Output - HI":T39, "Inputs":T38[], "Output Values":T39[], "Num. Inputs":i32, "Set Point":T39, "Inv.":bool[], "Inv. A":bool, "Inv. B":bool, "Input B":T38}
  T38 = typedef "DIO_selector.ctl" = i32
  T39 = typedef "output_value.ctl" = fxp<+/-,20,5>
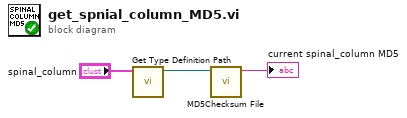
[diagram p0: block diagram]
diagram:
  n1 = call <vilib>:"Get Type Definition Path.vi"("Variant"="spinal_column") -> ("Type Definition Path"=w1:path)  [unwired: 9 in, 1 out]
  n2 = call <vilib>:"MD5Checksum File.vi"("Path"=w1) -> ("MD5 message-digest"=→"current spinal_column MD5":string)  [unwired: 9 in, 1 out]
